vi "Configure Dialog.vi"(8 "error in (no error)":errorcluster, 11 "Configure Arbitrary Sequence [SEQ] Msg.lvclass":refnum<class "Configure Arbitrary Sequence [SEQ] Msg.lvclass">) -> (0 "error out":errorcluster, 2 "Ok?":bool, 3 "Configure Arbitrary Sequence [SEQ] Msg.lvclass":refnum<class "Configure Arbitrary Sequence [SEQ] Msg.lvclass">)   [LabVIEW 2015, in "CS++Fgen.lvlib" / "Configure Arbitrary Sequence [SEQ] Msg.lvclass"]
uses:
  Configure Arbitrary Sequence [SEQ] Msg.lvclass
  Configure Arbitrary Sequence [SEQ] Msg.lvclass/Configure Arbitrary Sequence [SEQ] Msg.ctl
panel:
  in  "offset":dbl[unit]
  in  "gain":dbl
  in  "sequence handle":i32
  in  "channel name":string
  in  "Cancel Button":bool
  in  "OK Button":bool
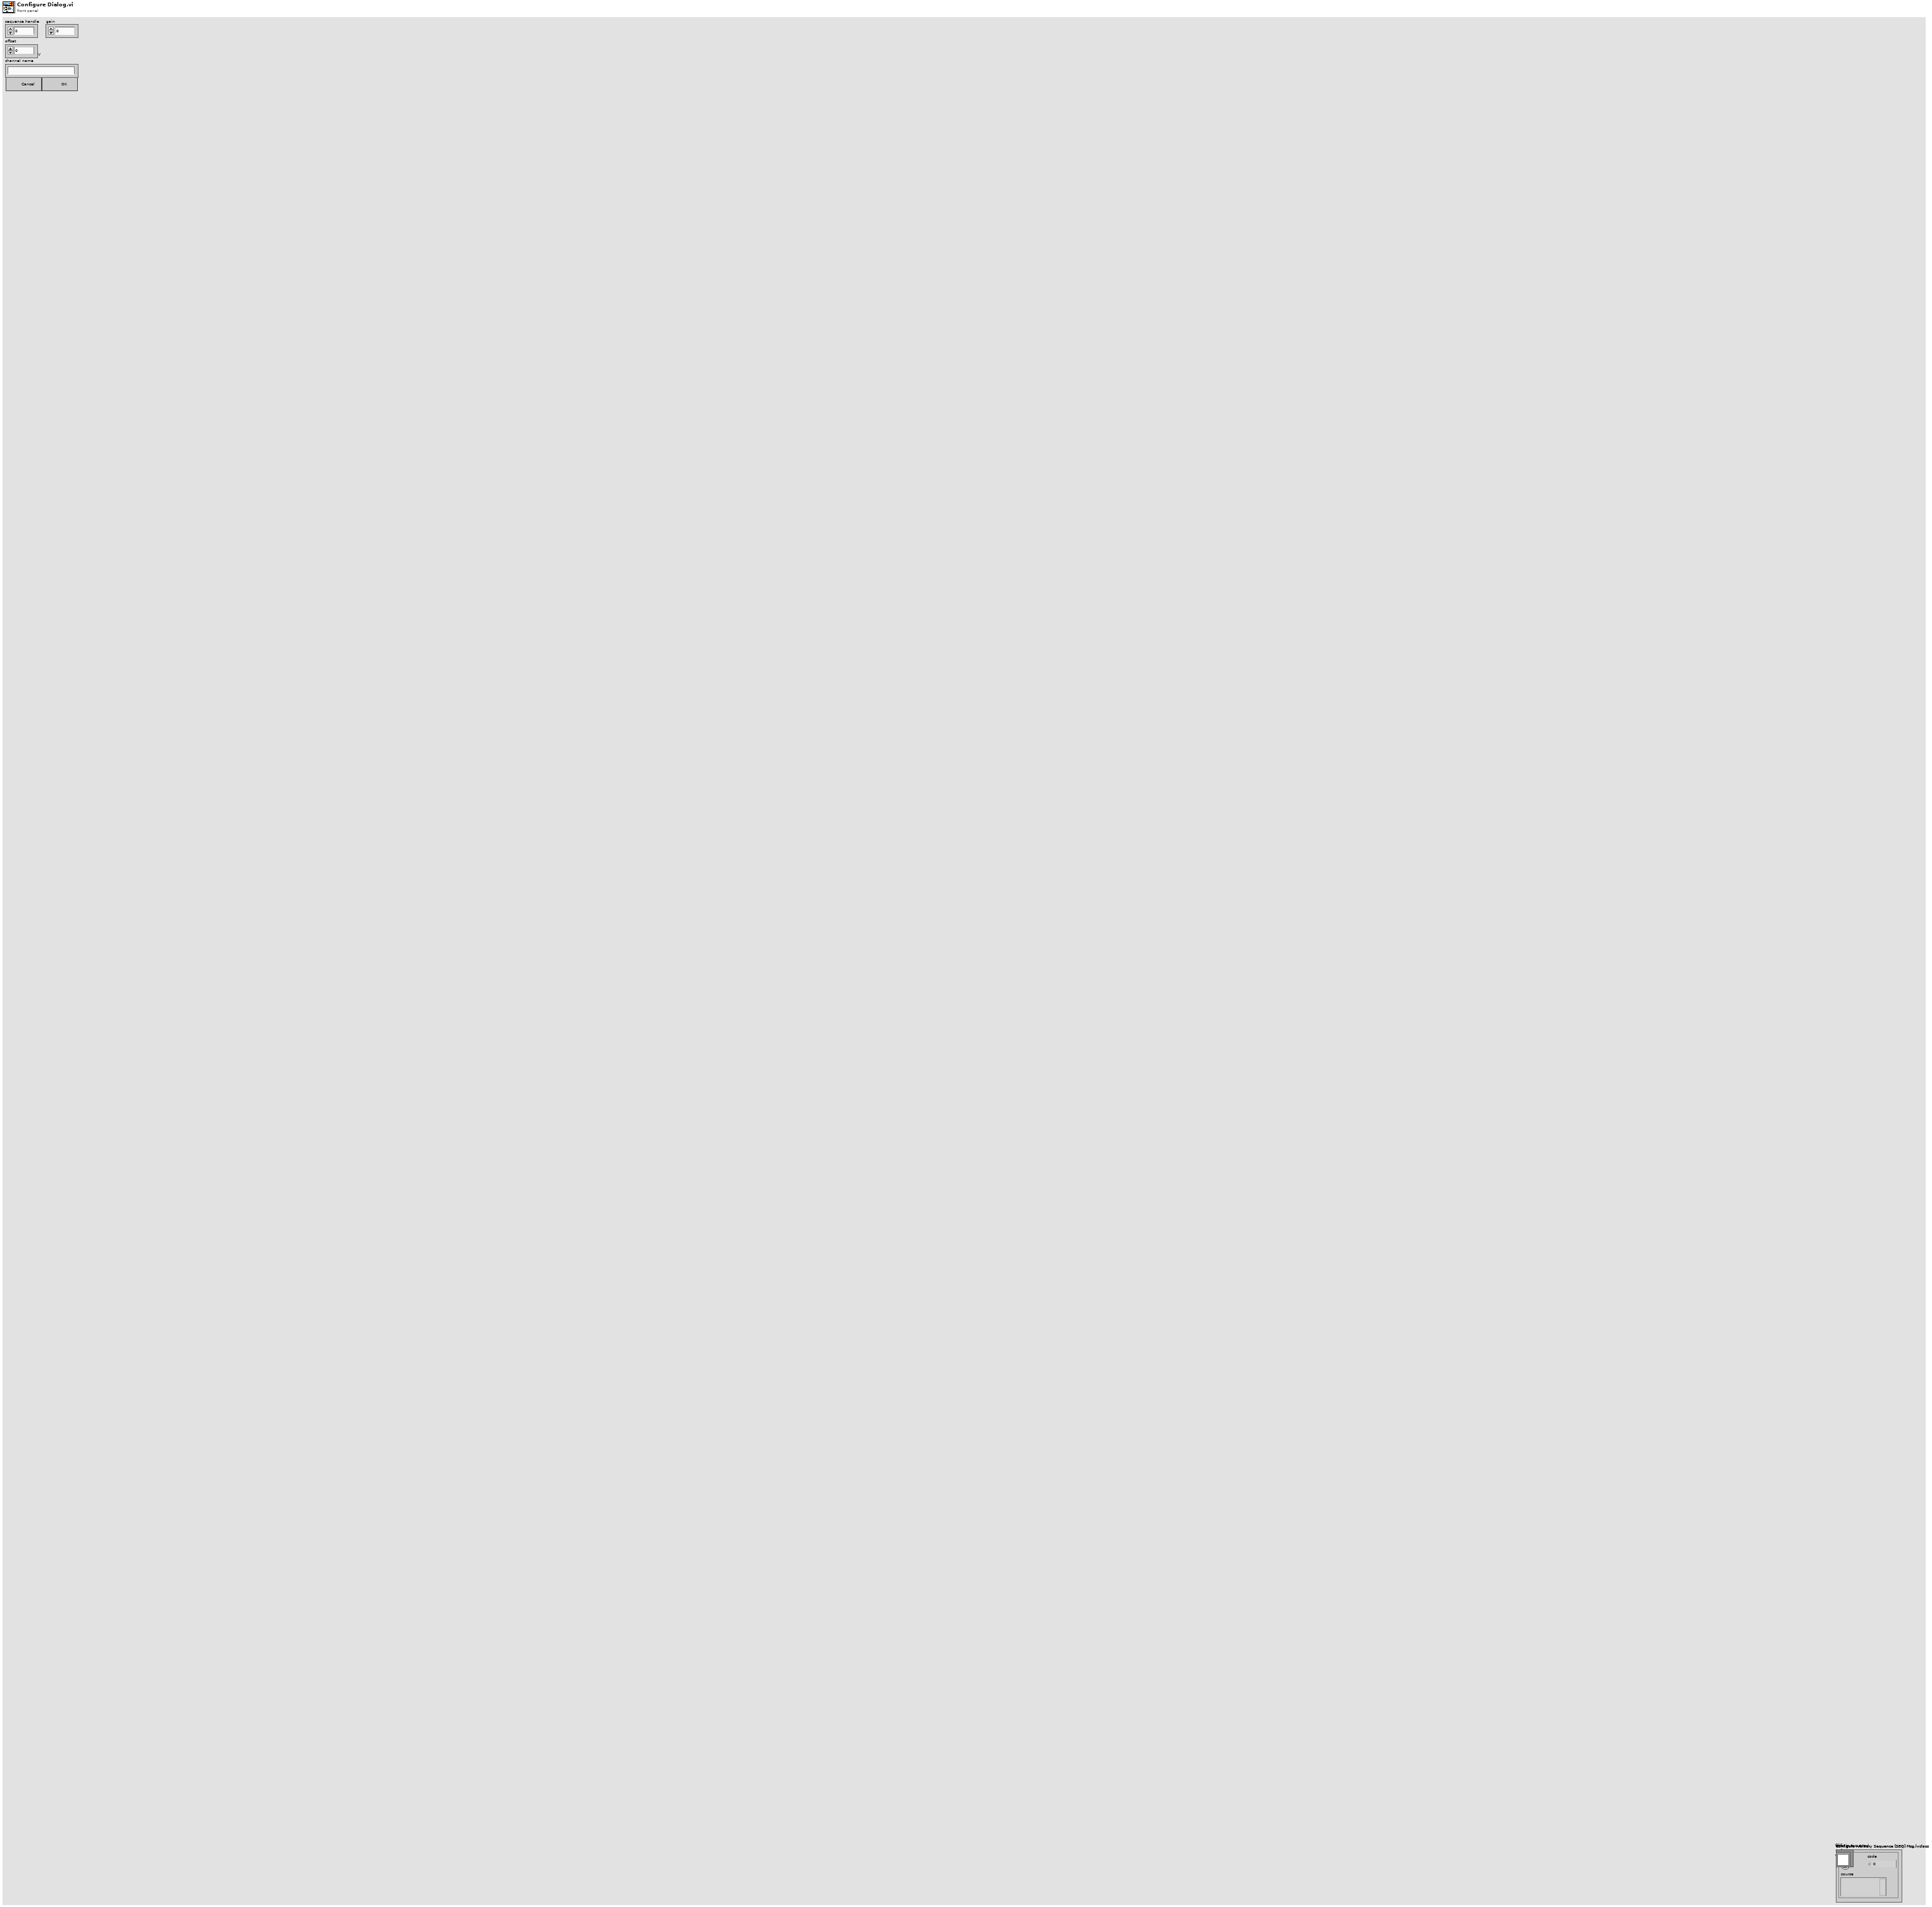
[diagram p1: front panel]
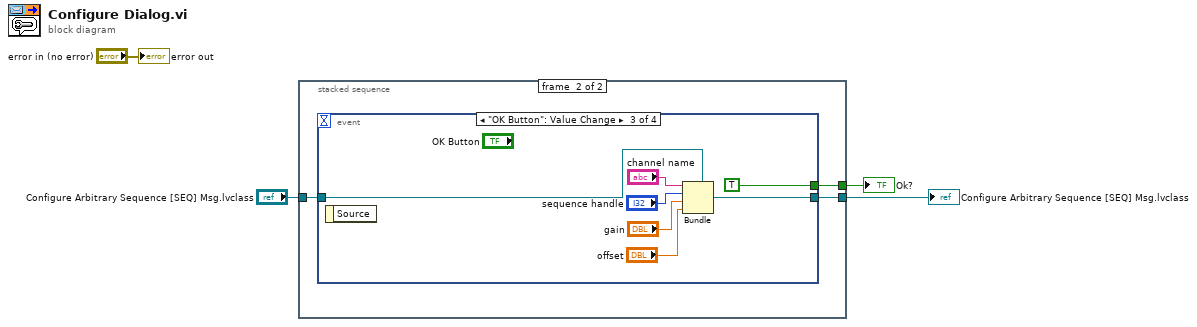
[diagram p0: block diagram]
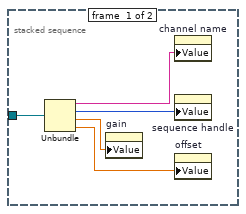
[diagram p2: hidden frame]
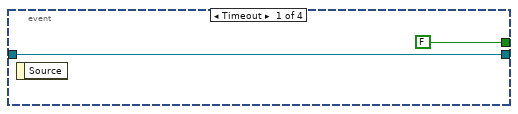
[diagram p3: hidden frame]
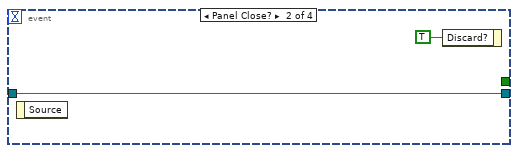
[diagram p4: hidden frame]
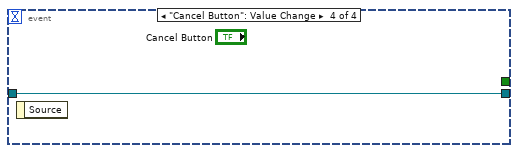
[diagram p5: hidden frame]
diagram:
  n1 = stacked-sequence {
    tunnel: [_ w12] -> w3
    tunnel: [_ w11] -> w2
    tunnel: "Configure Arbitrary Sequence [SEQ] Msg.lvclass" -> [w9 w10]
    frame #0 {
      n2 = Unbundle ("Seq0Unbundler")(w9) -> (w8:string, w7:i32, w6:dbl, w5:dbl[unit])
      n3 = property on="gain" class="DigNum (strict)"("Value"=w6) -> ()  [unwired: 2 in, 2 out]
      n4 = property on="channel name" class="Str"("Value"=w8) -> ()  [unwired: 2 in, 2 out]
      n5 = property on="sequence handle" class="DigNum (strict)"("Value"=w7) -> ()  [unwired: 2 in, 2 out]
      n6 = property on="offset" class="DigNum (strict)"("Value"=w5) -> ()  [unwired: 2 in, 2 out]
    }
    frame #1 {
      n7 = event shown="[2] \"OK Button\": Value Change" {
        selector: _ -> [_ _ _ _]
        dyn-events: _ -> [_ _ _ _]
        timeout: _ -> [_ _ _ _]
        tunnel: [w13 w15 w21 w24] -> w11
        tunnel: w10 -> [w13 w15 w23 w24]
        tunnel: [FALSE _ TRUE _] -> w12
        event Timeout {
          n8 = event-data() -> ()  [unwired: 1 in, 1 out]
        }
        event Panel Close? {
          n9 = event-data() -> ()  [unwired: 1 in, 1 out]
          n10 = event-data ("Event Filter Node")("Discard?"=TRUE) -> ()  [unwired: 1 in, 1 out]
        }
        event "OK Button": Value Change {
          n11 = event-data() -> ()  [unwired: 1 in, 1 out]
          n12 = Bundle ("Main-Bundler")(cluster=w23, "channel name", "sequence handle", "gain", "offset") -> (w21:refnum<class "Configure Arbitrary Sequence [SEQ] Msg.lvclass">)
        }
        event "Cancel Button": Value Change {
          n13 = event-data() -> ()  [unwired: 1 in, 1 out]
        }
      }
    }
  }
  "Ok?" <- w3
  "Configure Arbitrary Sequence [SEQ] Msg.lvclass" <- w2
  "error out" <- "error in (no error)"
